vi "arguments help.vi"() -> (3 "args help":string)   [LabVIEW 2013]
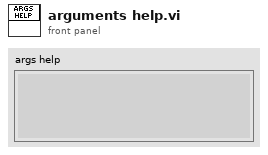
[diagram p1: front panel]
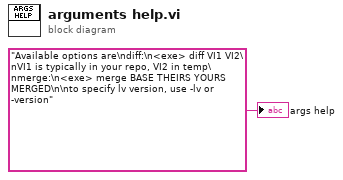
[diagram p0: block diagram]
diagram:
  "args help" <- "Available options are\ndiff:\n<exe> diff VI1 VI2\nVI1 is typically in your repo, VI2 in temp\nmerge:\n<exe> merge BASE THEIRS YOURS MERGED\n\nto specify lv version, use -lv or -version" ("args help")
